vi "Create_WF.vi"(8 "error in":errorcluster caption="entrée d'erreur", 11 "Scanning cluster":T1={"Nx"=4, "Ny"=4, "# Repetition"=1, "FOV_X (µm)"=100.0, "FOV_Y (µm)"=100.0, "Calib_X"=0.1, "Calib_Y"=0.1, "Center X (µm)"=50.0, "Center_Y (µm)"=50.0, "Bi-directionnal?"=FALSE} {"# Repetition" min=1 step=1; "Ny" min=1 step=1; "Nx" min=1 step=1}) -> (0 "error out":errorcluster caption="sortie d'erreur", 2 "Graphe":dbl[][](graph), 3 "2D table":dbl[][](array[numeric])=[[0.0, 3.333333333333333, 6.666666666666666, 10.0, 0.0, 3.333333333333333, 6.666666666666666, 10.0, 0.0, 3.333333333333333, 6.666666666666666, 10.0, 0.0, 3.333333333333333, 6.666666666666666, 10.0], [0.0, 0.0, 0.0, 0.0, 3.333333333333333, 3.333333333333333, 3.333333333333333, 3.333333333333333, 6.666666666666666, 6.666666666666666, 6.666666666666666, 6.666666666666666, 10.0, 10.0, 10.0, 10.0]])   [LabVIEW 2026]
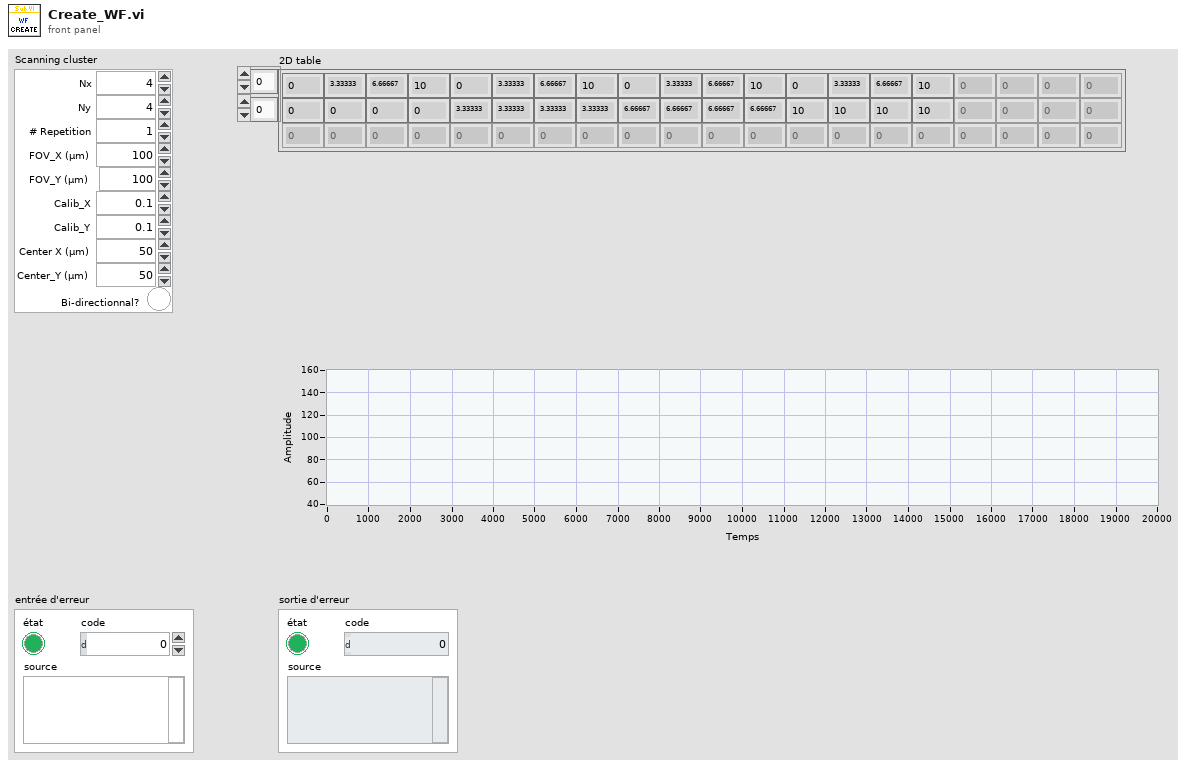
[diagram p1: front panel]
types:
  T1 = cluster{"Nx":u16, "Ny":u16, "# Repetition":u16, "FOV_X (µm)":dbl, "FOV_Y (µm)":dbl, "Calib_X":dbl, "Calib_Y":dbl, "Center X (µm)":dbl, "Center_Y (µm)":dbl, "Bi-directionnal?":bool}
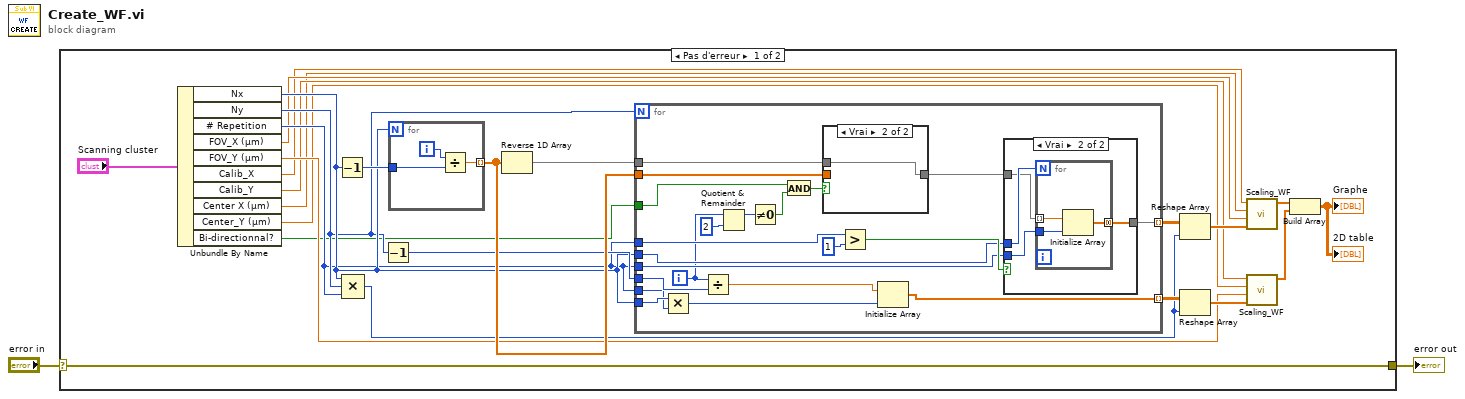
[diagram p0: block diagram]
diagram:
  n1 = case shown="Pas d'erreur" "error in" {
    selector: "error in" -> [w26 w61]
    tunnel: [w26 w61] -> w1
    frame No Error {
      n2 = Unbundle By Name("Scanning cluster") -> ("Nx"=w12:u16, "Ny"=w11:u16, "# Repetition"=w10:u16, "FOV_X (µm)"=w9:dbl, "FOV_Y (µm)"=w8:dbl, "Calib_X"=w7:dbl, "Calib_Y"=w6:dbl, "Center X (µm)"=w5:dbl, "Center_Y (µm)"=w4:dbl, "Bi-directionnal?"=w3:bool)
      n3 = Decrement(x=w12) -> (x-1=w25:u16)
      n4 = Compound Arithmetic op=MULTIPLY(w12, w11, w10) -> (w19:u16)
      n5 = Decrement(x=w11) -> (x-1=w22:u16)
      n6 = for {
        N: w12 -> [_]
        tunnel: w25 -> [w59]
        tunnel: [w58] -> w24 mode=indexing
        i -> [w60]
        n7 = Divide(x=w60, y=w59) -> (x/y=w58:dbl)
      }
      n8 = Reverse 1D Array(array=w24) -> (reversed array=w23:dbl[])
      n9 = for {
        N: w11 -> [_]
        tunnel: w3 -> [w45]
        tunnel: w24 -> [w42]
        tunnel: w23 -> [w41]
        tunnel: w10 -> [w40]
        tunnel: w12 -> [w36]
        tunnel: w10 -> [w35]
        tunnel: w22 -> [w34]
        tunnel: w12 -> [w31]
        tunnel: w10 -> [w30]
        tunnel: [w28] -> w21 mode=indexing
        tunnel: [w27] -> w20 mode=indexing
        i -> [w33]
        n10 = Multiply(x=w31, y=w30) -> (x*y=w29:u16)
        n11 = Divide(x=w33, y=w34) -> (x/y=w32:dbl)
        n12 = Quotient & Remainder(x=w33, y=2) -> (x-y*floor(x/y)=w46:i32)  [unwired: 1 out]
        n13 = Not Equal To 0?(x=w46) -> (x != 0?=w47:bool)
        n14 = And(x=w45, y=w47) -> (x .and. y?=w44:bool)
        n15 = case shown="Vrai" w44 {
          tunnel: [w56 w57] -> w37
          tunnel: w42 -> [w56 _]
          tunnel: w41 -> [_ w57]
          frame False {
          }
          frame True {
          }
        }
        n16 = Greater?(x=w40, y=u16 1) -> (0:w38:bool)
        n17 = Initialize Array(w32, w29) -> (w27:dbl[])
        n18 = case shown="Vrai" w38 {
          tunnel: [w48 w49] -> w28
          tunnel: w37 -> [w48 w51]
          tunnel: w36 -> [_ w52]
          tunnel: w35 -> [_ w50]
          frame False {
          }
          frame True {
            n19 = for {
              N: w52 -> [_]
              tunnel: w51 -> [w55] mode=indexing
              tunnel: w50 -> [w54]
              tunnel: [w53] -> w49 mode=concatenating
              n20 = Initialize Array(w55, w54) -> (w53:dbl[])
            }
          }
        }
      }
      n21 = Reshape Array(w21, w19) -> (w18:dbl[])
      n22 = Reshape Array(w20, w19) -> (w16:dbl[])
      n23 = call "Scaling_WF.vi"("Axis_unit_1D"=w18, "FOV_Axis (µm)"=w9, "Center Axis (µm)"=w5, "Calib_Axis"=w7) -> ("Axis_volts"=w17:dbl[])  [unwired: 7 in]
      n24 = call "Scaling_WF.vi"("Axis_unit_1D"=w16, "FOV_Axis (µm)"=w8, "Center Axis (µm)"=w4, "Calib_Axis"=w6) -> ("Axis_volts"=w15:dbl[])  [unwired: 7 in]
      n25 = Build Array(w17, w15) -> (→"2D table" →"Graphe":dbl[][])
    }
    frame Error {
    }
  }
  "error out" <- w1
